vi "Pre Init Controls.vi"(6 "find list":string[](array[string]), 7 "Cluster Refernz Cluster":T1, 8 "Fehler (Eingang, kein Fehler)":errorcluster, 9 "Connect Referenz":refnum<vi>, 10 "Str Referenz":refnum<vi>, 11 "Ring (Eingang)":refnum<vi>) -> (0 "Fehler (Ausgang)":errorcluster, 3 "empty?":bool)   [LabVIEW 2020, in "Linearisierung v2.lvlib" / "Gasteiler.lvlib" / "HovaCAL_Interface.lvlib" / "Helper.lvlib"]
uses:
  Helper.lvlib
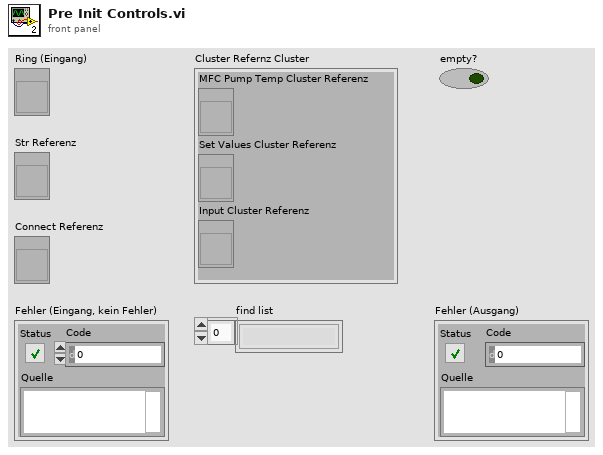
[diagram p1: front panel]
types:
  T1 = cluster{"MFC Pump Temp Cluster Referenz":refnum<vi>, "Set Values Cluster Referenz":refnum<vi>, "Input Cluster Referenz":refnum<vi>}
  T2 = enum8{"Enabled", "Disabled", "Disabled and Grayed Out"}
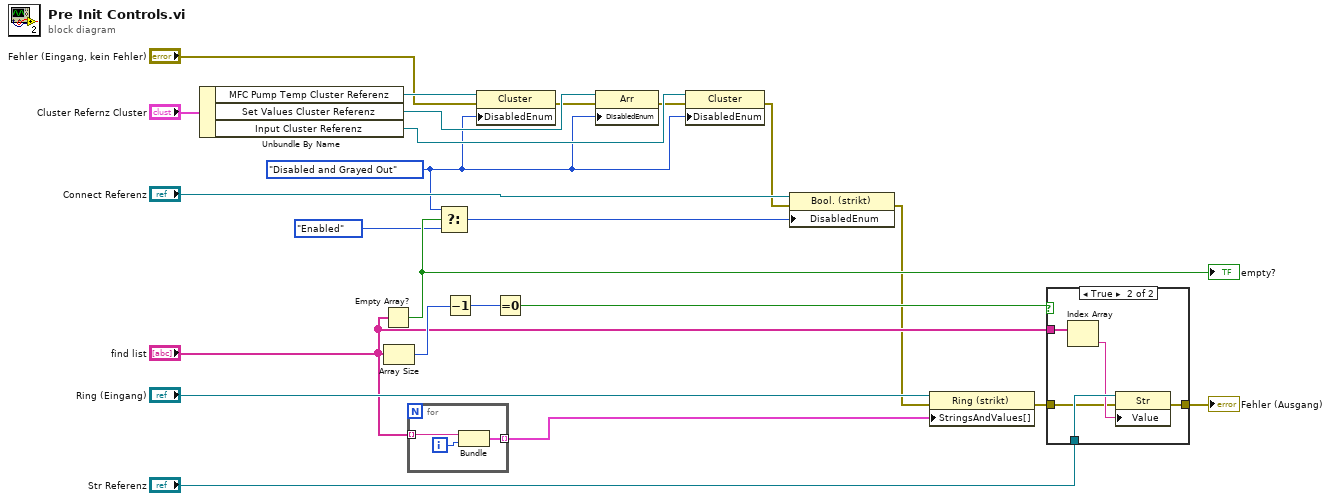
[diagram p0: block diagram]
diagram:
  w7 = T2."Disabled and Grayed Out" ("Deaktiviert")
  n1 = Unbundle By Name("Cluster Refernz Cluster") -> ("MFC Pump Temp Cluster Referenz"=w10:refnum<vi>, "Set Values Cluster Referenz"=w9:refnum<vi>, "Input Cluster Referenz"=w8:refnum<vi>)
  n2 = Empty Array?(array="find list") -> (empty?=w21:bool)
  "empty?" <- w21
  n3 = Array Size(array="find list") -> (size(s)=w22:i32)
  n4 = for {
    tunnel: "find list" -> [w26] mode=indexing
    tunnel: [w24] -> w20 mode=indexing
    i -> [w25]
    n5 = Bundle(w26, w25) -> (w24:cluster{string, i32})  [unwired: 1 in]
  }
  n6 = Select(t=w7, s=w21, f=T2."Enabled" ("Deaktiviert")) -> (s? t:f=w13:T2)
  n7 = Decrement(x=w22) -> (x-1=w23:i32)
  n8 = property class="Cluster"(reference=w10, error in="Fehler (Eingang, kein Fehler)", "DisabledEnum"=w7) -> (error out=w5:errorcluster)  [unwired: 1 out]
  n9 = Equal To 0?(x=w23) -> (x = 0?=w2:bool)
  n10 = property class="Arr"(reference=w9, error in=w5, "DisabledEnum"=w7) -> (error out=w4:errorcluster)  [unwired: 1 out]
  n11 = property class="Cluster"(reference=w8, error in=w4, "DisabledEnum"=w7) -> (error out=w3:errorcluster)  [unwired: 1 out]
  n12 = property class="Bool. (strikt)"(reference="Connect Referenz", error in=w3, "DisabledEnum"=w13) -> (error out=w1:errorcluster)  [unwired: 1 out]
  n13 = property on="Eigenschaftsknoten" class="Ring (strikt)"(reference="Ring (Eingang)", error in=w1, "StringsAndValues[]"=w20) -> (error out=w16:errorcluster)  [unwired: 1 out]
  n14 = case shown="True" w2 {
    tunnel: "Str Referenz" -> [_ w32]
    tunnel: "find list" -> [_ w31]
    tunnel: w16 -> [w27 w29]
    tunnel: [w27 w28] -> w15
    frame False {
    }
    frame True {
      n15 = Index Array(array=w31) -> (element=w30:string)  [unwired: 1 in]
      n16 = property on="Eigenschaftsknoten" class="Str"(reference=w32, error in=w29, "Value"=w30) -> (error out=w28:errorcluster)  [unwired: 1 out]
    }
  }
  "Fehler (Ausgang)" <- w15
